vi "Logger_Loop.vi"(11 "TDMS DevRef In":T1) -> ()   [LabVIEW 2017]
uses:
  <userlib>/836-Library/System/TDMS_V2/Support/TDMS_DevRef.ctl
  <userlib>/836-Library/System/TDMS_V2/Support/Logging_Settings.ctl
  <userlib>/836-Library/System/TDMS_V2/Support/Group_FIFO_Config.ctl
  <userlib>/836-Library/System/TDMS_V2/Support/Channel_FIFO_Config.ctl
  <vilib>/Platform/TimedLoop/XDataNode/timing_clust.ctl
  <vilib>/Platform/TimedLoop/XDataNode/nitl_modes.ctl
  <vilib>/Platform/TimedLoop/XDataNode/wakeup.ctl
  <vilib>/platform/TimedLoop/XDataNode/XDataNode.xnode
  <vilib>/Platform/TimedLoop/XDataNode/XDNodeRunTimeDep.lvlib
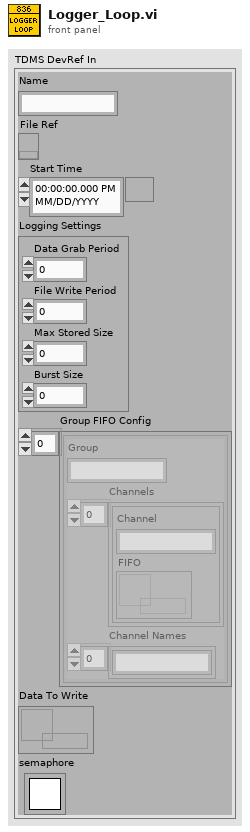
[diagram p1: front panel]
types:
  T1 = typedef "TDMS_DevRef.ctl" = cluster{"Name":string, "File Ref":refnum<k34>, "Start Time":timestamp, "Logging Settings":T2, "Group FIFO Config":T3[], "Data To Write":refnum<data-value>, "semaphore":T5}
  T2 = typedef "Logging_Settings.ctl" = cluster{"Data Grab Period":dbl, "File Write Period":dbl, "Max Stored Size":dbl, "Burst Size":dbl}
  T3 = typedef "Group_FIFO_Config.ctl" = cluster{"Group":string, "Channels":T4[], "Channel Names":string[]}
  T4 = typedef "Channel_FIFO_Config.ctl" = cluster{"Channel":string, "FIFO":refnum<k33>}
  T5 = typedef "Semaphore RefNum" = refnum<k1>
  T6 = typedef "XDNodeRunTimeDep.lvlib/timing_clust.ctl" = cluster{"Expected End [f-1]":u64, "Actual End [f-1]":u64, "Finished Late? [f-1]":bool, "Expected End [i-1]":u64, "Actual End [i-1]":u64, "Finished Late? [i-1]":bool, "Expected Start [i]":u64, "Actual Start [i]":u64, "Expected Start [f]":u64, "Actual Start [f]":u64, "Source Name":string, "Structure Name":string, "Period":i64, "Deadline":i64, "Offset":i64, "Start":i64, "Priority":i32, "Timeout":i32, "Mode":T7, "Wakeup Reason":T8, "Error":errorcluster, "Source Type":string, "Secondary Source Type":string, "Global End Time":u64, "Global Start Time":u64, "Frame Duration":u64, "Iteration Duration":u64, "Assigned CPU":i32, "I/O Scan Engine Mode":u32}
  T7 = typedef "XDNodeRunTimeDep.lvlib/nitl_modes.ctl" = enum32{"No Change", "Process missed periods, maintain original phase", "Discard missed periods, maintain original phase", "Process missed periods, ignore original phase", "Discard missed periods, ignore original phase"}
  T8 = typedef "XDNodeRunTimeDep.lvlib/wakeup.ctl" = enum32{"Normal", "Aborted", "Asynchronous wakeup", "Timing source error", "Timed loop error", "Timeout"}
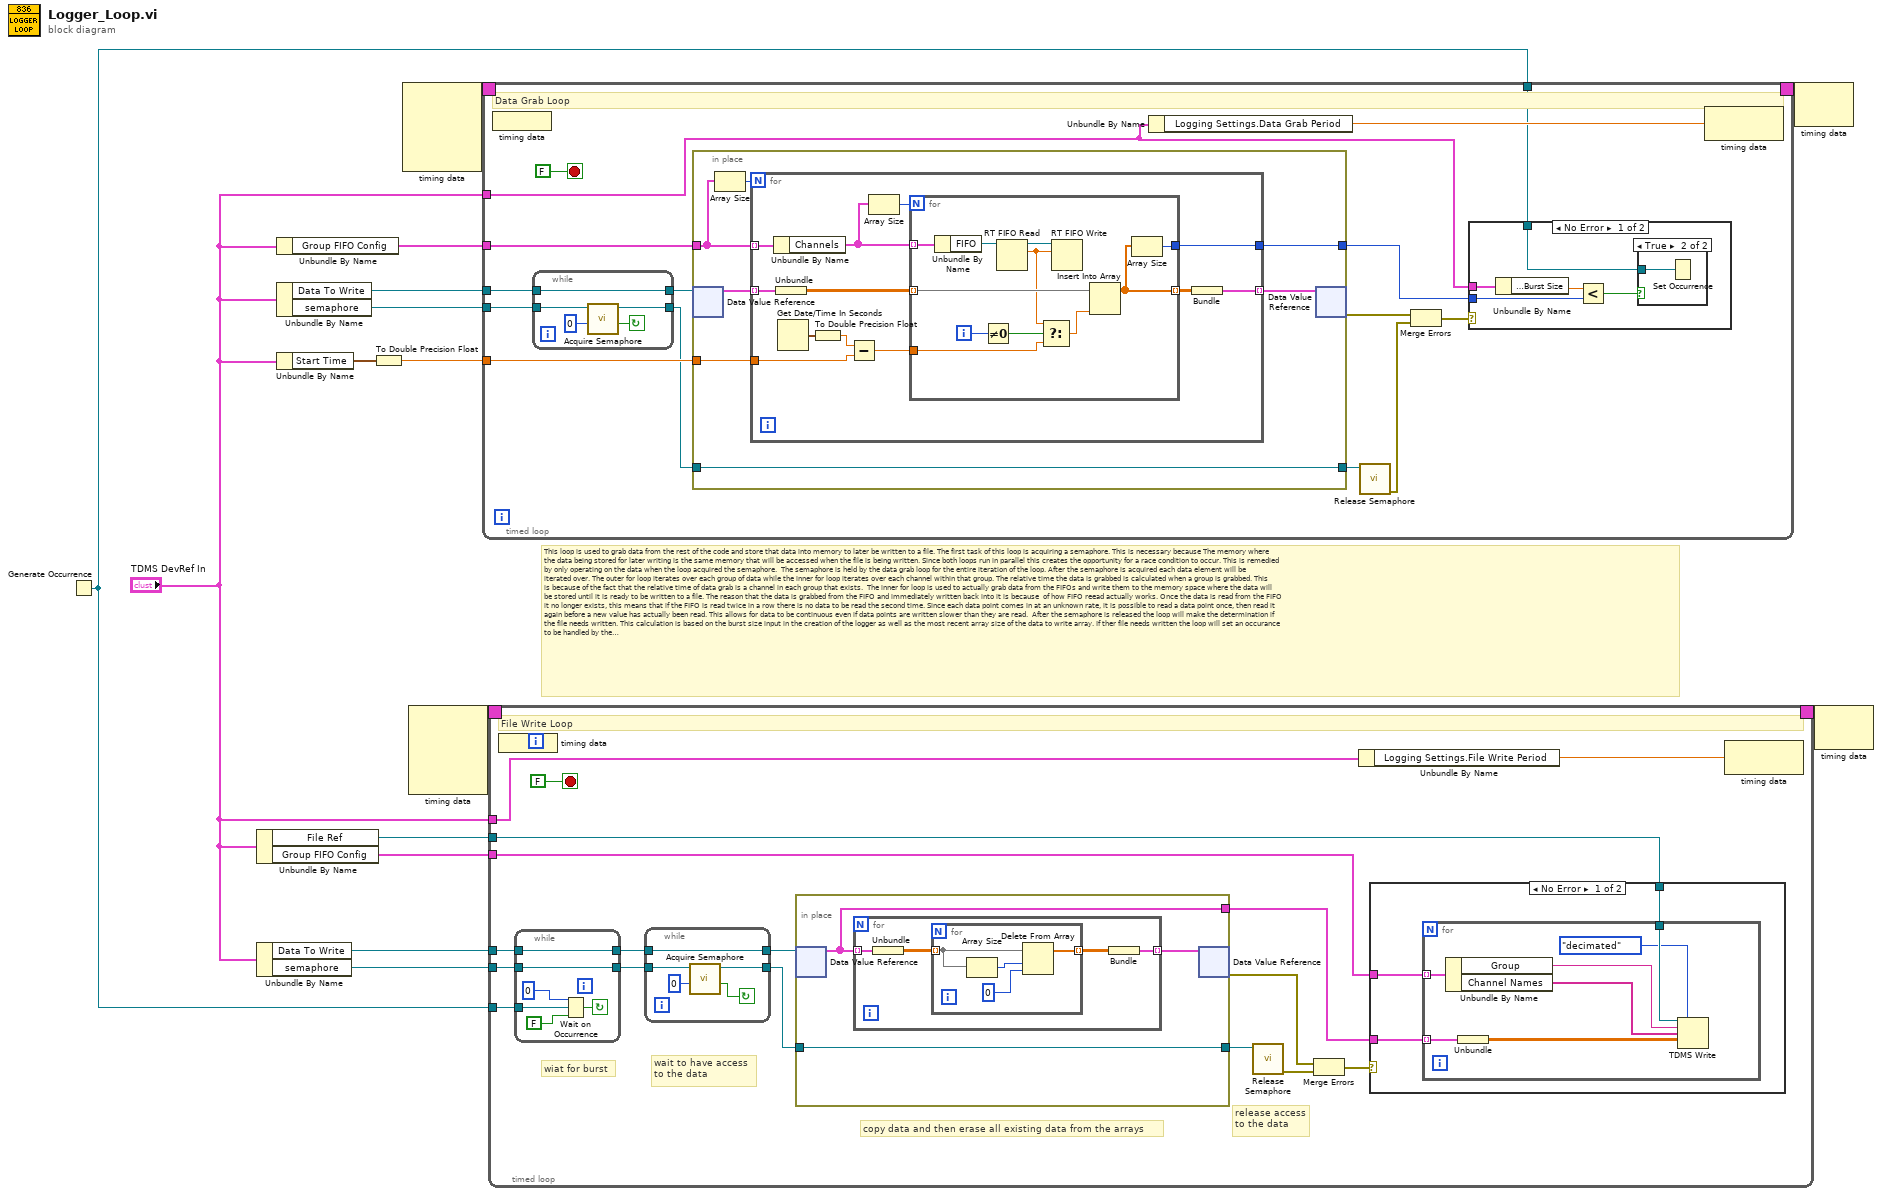
[diagram p0: block diagram]
diagram:
  # "This loop is used to grab data from the rest of the code and store that data into memory to later be written to a file. The first task of this loop is acquiring a semaphore. This is necessary because The memory where\nthe data being stored for later writing is the same memory that will be accessed when the file is being written. Since both loops run in parallel this creates the opportunity for a race condition to occur. This is remedied\nby only operating on the data when the loop acquired the semaphore.  The semaphore is held by the data grab loop for the entire iteration of the loop. After the semaphore is acquired each data element will be\niterated over. The outer for loop iterates over each group of data while the inner for loop iterates over each channel within that group. The relative time the data is grabbed is calculated when a group is grabbed. This\nis because of the fact that the relative time of data grab is a channel in each group that exists.  The inner for loop is used to actually grab data from the FIFOs and write them to the memory space where the data will\nbe stored until it is ready to be written to a file. The reason that the data is grabbed from the FIFO and immediately written back into it is because  of how FIFO reead actually works. Once the data is read from the FIFO\nit no longer exists, this means that if the FIFO is read twice in a row there is no data to be read the second time. Since each data point comes in at an unknown rate, it is possible to read a data point once, then read it\nagain before a new value has actually been read. This allows for data to be continuous even if data points are written slower than they are read.  After the semaphore is released the loop will make the determination if\nthe file needs written. This calculation is based on the burst size input in the creation of the logger as well as the most recent array size of the data to write array. If ther file needs written the loop will set an occurance\nto be handled by the File Write Loop."
  n1 = Generate Occurrence() -> (w4:refnum<k4>)
  n2 = Unbundle By Name("TDMS DevRef In") -> ("File Ref"=w2:refnum<k34>, "Group FIFO Config"=w1:T3[])
  n3 = Unbundle By Name("TDMS DevRef In") -> ("Data To Write"=w6:refnum<data-value>, "semaphore"=w5:T5)
  n4 = Unbundle By Name("TDMS DevRef In") -> ("Group FIFO Config"=w9:T3[])
  n5 = Unbundle By Name("TDMS DevRef In") -> ("Data To Write"=w13:refnum<data-value>, "semaphore"=w12:T5)
  n6 = Unbundle By Name("TDMS DevRef In") -> ("Start Time"=w11:timestamp)
  n7 = To Double Precision Float(number=w11) -> (double precision float=w10:dbl)
  n8 = node-c288() -> (w15:T6)  [unwired: 4 in]
  n9 = node-c288() -> (w8:T6)  [unwired: 4 in]
  n10 = timed-loop {
    timing: w15 -> [_]
    timing-out: [_] -> w14
    tunnel: "TDMS DevRef In" -> [w17]
    tunnel: w13 -> [w29]
    tunnel: w12 -> [w24]
    tunnel: w10 -> [w27]
    tunnel: w9 -> [w25]
    tunnel: w4 -> [w16]
    stop <- FALSE stop-if-true
    # "Data Grab Loop"
    n11 = node-c288() -> ()  [unwired: 1 in]
    n12 = while {
      tunnel: w24 -> [w71]
      tunnel: w29 -> [w68]
      tunnel: [w68] -> w26
      tunnel: [w67] -> w23
      stop <- w70 continue-if-true
      n13 = call <vilib>:"Acquire Semaphore.vi"("ms timeout (-1)"=0, "semaphore"=w71) -> ("timed out"=w70:bool, "semaphore out"=w67:T5)  [unwired: 3 in, 1 out]
    }
    n14 = in-place {
      in-place-border: w27 -> [w42]
      in-place-border: w25 -> [w37]
      in-place-border: w23 -> [w40]
      in-place-border: [w40] -> w22
      in-place-border: [w39] -> w18
      n15 = in-place-dvr #1(w26) -> (w43:cluster{dbl[][]}[])  [unwired: 1 out]
      n16 = Array Size(array=w37) -> (size(s)=w38:i32)
      n17 = for {
        N: w38 -> [_]
        tunnel: w43 -> [w51] mode=indexing
        tunnel: w37 -> [w55] mode=indexing
        tunnel: w42 -> [w52]
        tunnel: [w47] -> w41 mode=indexing
        tunnel: [w46] -> w39
        n18 = Unbundle By Name(w55) -> ("Channels"=w44:T4[])
        n19 = Unbundle(w51) -> (w50:dbl[][])
        n20 = Get Date/Time In Seconds() -> (seconds since 1Jan1904=w54:timestamp)
        n21 = To Double Precision Float(number=w54) -> (double precision float=w53:dbl)
        n22 = Subtract(x=w53, y=w52) -> (x-y=w49:dbl)
        n23 = Array Size(array=w44) -> (size(s)=w45:i32)
        n24 = for {
          N: w45 -> [_]
          tunnel: w50 -> [w63] mode=indexing
          tunnel: w44 -> [w66] mode=indexing
          tunnel: w49 -> [w60]
          tunnel: [w57] -> w48 mode=indexing
          tunnel: [w56] -> w46
          i -> [w61]
          n25 = Unbundle By Name(w66) -> ("FIFO"=w65:refnum<k33>)
          n26 = Not Equal To 0?(x=w61) -> (x != 0?=w62:bool)
          n27 = RT FIFO Read(0:w65) -> (8:w64:refnum<k33>, 9:w59:dbl)  [unwired: 3 in, 3 out]
          n28 = Select(t=w59, s=w62, f=w60) -> (s? t:f=w58:dbl)
          n29 = RT FIFO Write(0:w64, 1:w59) -> ()  [unwired: 3 in, 4 out]
          n30 = Insert Into Array(array=w63, new element=w58) -> (w57:dbl[])  [unwired: 1 in]
          n31 = Array Size(array=w57) -> (size(s)=w56:i32)
        }
        n32 = Bundle(w48) -> (w47:cluster{dbl[][]})  [unwired: 1 in]
      }
      n33 = in-place-dvr #1(w41) -> (w20:errorcluster)  [unwired: 1 out]
    }
    n34 = Unbundle By Name(w17) -> ("Logging Settings.Data Grab Period"=w30:dbl)
    n35 = call <vilib>:"Release Semaphore.vi"("semaphore"=w22) -> ("error out"=w21:errorcluster)  [unwired: 5 in, 1 out]
    n36 = Merge Errors(w20, w21) -> (w19:errorcluster)
    n37 = case shown="No Error" w19 {
      tunnel: w18 -> [w35 _]
      tunnel: w17 -> [w34 _]
      tunnel: w16 -> [w31 _]
      frame No Error {
        n38 = Unbundle By Name(w34) -> ("Logging Settings.Burst Size"=w33:dbl)
        n39 = Less?(x=w33, y=w35) -> (x < y?=w32:bool)
        n40 = case shown="True" w32 {
          tunnel: w31 -> [_ w36]
          frame False {
          }
          frame True {
            n41 = Set Occurrence(w36) -> ()
          }
        }
      }
      frame Error {
      }
    }
    n42 = node-c288(w30) -> ()  [unwired: 1 out]
  }
  n43 = timed-loop {
    timing: w8 -> [_]
    timing-out: [_] -> w7
    tunnel: "TDMS DevRef In" -> [w92]
    tunnel: w6 -> [w88]
    tunnel: w5 -> [w89]
    tunnel: w4 -> [w90]
    tunnel: w2 -> [w78]
    tunnel: w1 -> [w77]
    stop <- FALSE stop-if-true
    # "release access\nto the data"
    # "copy data and then erase all existing data from the arrays"
    # "wait to have access\nto the data"
    # "wiat for burst"
    # "File Write Loop"
    n44 = node-c288() -> ()  [unwired: 1 in]
    n45 = while {
      tunnel: w90 -> [w124]
      tunnel: [w120] -> w87
      tunnel: w89 -> [w120]
      tunnel: [w119] -> w86
      tunnel: w88 -> [w119]
      stop <- w121 continue-if-true
      n46 = Wait on Occurrence(1:FALSE ("ignore previous (T)"), 2:w124, 3:0 ("ms timeout (-1)")) -> (0:w121:bool)
    }
    n47 = while {
      tunnel: w87 -> [w118]
      tunnel: [w115] -> w84
      tunnel: [w114] -> w85
      tunnel: w86 -> [w114]
      stop <- w116 continue-if-true
      n48 = call <vilib>:"Acquire Semaphore.vi"("ms timeout (-1)"=0, "semaphore"=w118) -> ("timed out"=w116:bool, "semaphore out"=w115:T5)  [unwired: 3 in, 1 out]
    }
    n49 = in-place {
      in-place-border: [w105] -> w79
      in-place-border: w84 -> [w103]
      in-place-border: [w103] -> w83
      n50 = in-place-dvr #2(w85) -> (w105:cluster{dbl[][]}[])  [unwired: 1 out]
      n51 = for {
        tunnel: w105 -> [w109] mode=indexing
        tunnel: [w106] -> w104 mode=indexing
        n52 = Unbundle(w109) -> (w108:dbl[][])
        n53 = for {
          tunnel: w108 -> [w111] mode=indexing
          tunnel: [w110] -> w107 mode=indexing
          n54 = Array Size(array=w111) -> (size(s)=w112:i32)
          n55 = Delete From Array(array=w111, length=w112, index=0) -> (array with subset deleted=w110:dbl[])  [unwired: 1 out]
        }
        n56 = Bundle(w107) -> (w106:cluster{dbl[][]})  [unwired: 1 in]
      }
      n57 = in-place-dvr #2(w104) -> (w81:errorcluster)  [unwired: 1 out]
    }
    n58 = call <vilib>:"Release Semaphore.vi"("semaphore"=w83) -> ("error out"=w82:errorcluster)  [unwired: 5 in, 1 out]
    n59 = Merge Errors(w81, w82) -> (w80:errorcluster)
    n60 = Unbundle By Name(w92) -> ("Logging Settings.File Write Period"=w91:dbl)
    n61 = case shown="No Error" w80 {
      tunnel: w79 -> [w95 _]
      tunnel: w78 -> [w94 _]
      tunnel: w77 -> [w93 _]
      frame No Error {
        n62 = for {
          tunnel: w95 -> [w99] mode=indexing
          tunnel: w94 -> [w100]
          tunnel: w93 -> [w102] mode=indexing
          n63 = Unbundle By Name(w102) -> ("Group"=w101:string, "Channel Names"=w96:string[])
          n64 = Unbundle(w99) -> (w98:dbl[][])
          n65 = TDMS Write(0:w100, 1:enum16{"decimated", "interleaved"}."decimated" ("data layout (0:decimated)"), 5:w101, 7:w96, 9:w98) -> ()  [unwired: 1 in, 4 out]
        }
      }
      frame Error {
      }
    }
    n66 = node-c288(w91) -> ()  [unwired: 1 out]
  }
  n67 = node-c288(w14) -> ()  [unwired: 1 out]
  n68 = node-c288(w7) -> ()  [unwired: 1 out]
